vi "Auton Select.vi"(9 "Select Previous":bool, 10 "Select Next":bool, 11 "Script Folder Path":string) -> (0 "error out":errorcluster, 1 "filenames":string[](array[string]), 2 "Selected Script":string, 3 "Script Path":string)   [LabVIEW 2015]
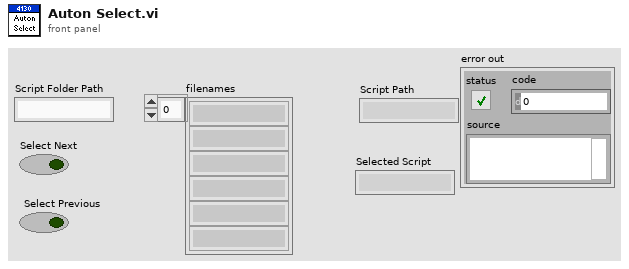
[diagram p1: front panel]
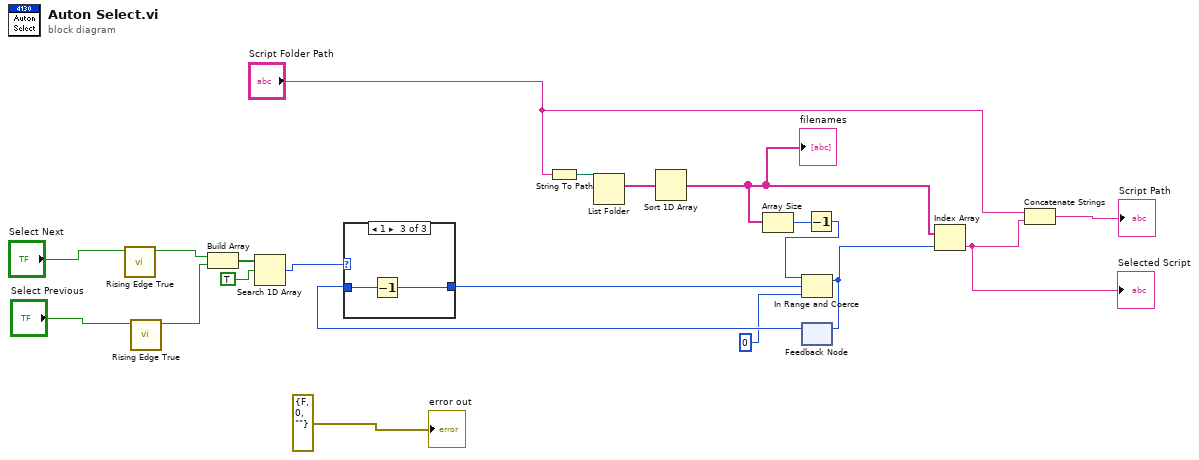
[diagram p0: block diagram]
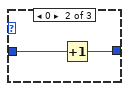
[diagram p3: hidden frame]
diagram:
  n1 = call "Rising Edge True.vi"("Input"="Select Next") -> ("Output"=w19:bool)  [unwired: 10 in]
  n2 = call "Rising Edge True.vi"("Input"="Select Previous") -> ("Output"=w20:bool)  [unwired: 10 in]
  n3 = Build Array(w19, w20) -> (w13:bool[])
  n4 = Search 1D Array(1D array=w13, element=TRUE) -> (index of element=w15:i32)  [unwired: 1 in]
  n5 = String To Path(string="Script Folder Path") -> (path=w3:path)
  n6 = List Folder(path=w3) -> (filenames=w6:string[])  [unwired: 3 in, 3 out]
  n7 = Sort 1D Array(array=w6) -> (sorted array=w2:string[])
  "filenames" <- w2
  n8 = Array Size(array=w2) -> (size(s)=w4:i32)
  n9 = feedback #1() -> (w16:i32)  [unwired: 1 in]
  n10 = case shown="1" w15 {
    tunnel: w16 -> [w21 w23 w25]
    tunnel: [w21 w22 w24] -> w17
    frame -1, Default {
    }
    frame 0 {
      n11 = Increment(x=w23) -> (x+1=w22:i32)
    }
    frame 1 {
      n12 = Decrement(x=w25) -> (x-1=w24:i32)
    }
  }
  n13 = Decrement(x=w4) -> (x-1=w5:i32)
  n14 = In Range and Coerce(upper limit=w5, x=w17, lower limit=0 ("datalog type")) -> (coerced(x)=w9:i32)  [unwired: 1 out]
  n15 = feedback-in #1(w9) -> ()
  n16 = Index Array(array=w2, index=w9) -> (element=w7:string)
  "Selected Script" <- w7
  n17 = Concatenate Strings("Script Folder Path", w7) -> (→"Script Path":string)
  "error out" <- errorcluster {"status"=FALSE, "code"=0, "source"=""} ("error constant")
